vi "Populate Ctrl.vi"(8 "error in (no error)":errorcluster, 11 "Text Field in":refnum<class "Text Field.lvclass">) -> (0 "error out":errorcluster, 3 "Text Field out":refnum<class "Text Field.lvclass">)   [LabVIEW 2020, in "Basic Fields.lvlib" / "Text Field.lvclass"]
uses:
  Text Field.lvclass
  Basic Fields/Basic Field Class/Ctrl Refnum Column.lvclass
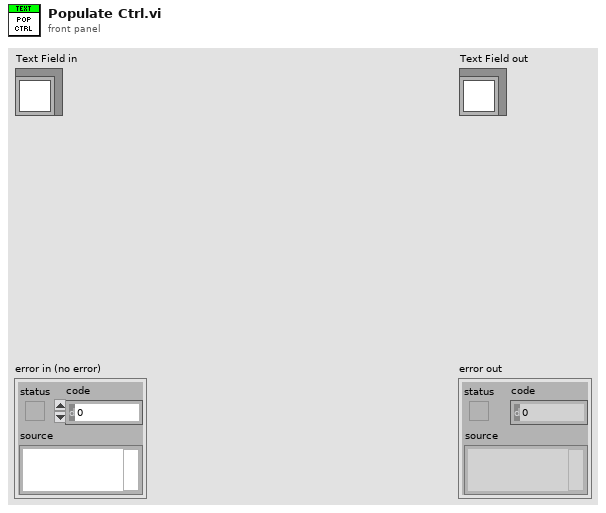
[diagram p1: front panel]
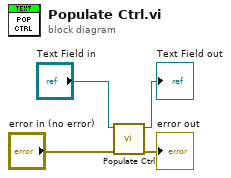
[diagram p0: block diagram]
diagram:
  n1 = call-parent "Populate Ctrl.vi"("error in (no error)"="error in (no error)", "Ctrl Refnum Column in"="Text Field in") -> ("error out"=→"error out":errorcluster, "Ctrl Refnum Column out"=→"Text Field out":refnum<class "Text Field.lvclass">)  [unwired: 8 in]
